vi "HapticSTM-Demod.vi"() -> ()   [LabVIEW 2019]
uses:
  Program Files/National Instruments/LabVIEW 2019/user.lib/HapticSTM/HapticSTM.lvlib
panel:
  out "Numeric":i32
  in  "Signal":u16(ring) items=["Z Val", "Demod", "AFM"]
  in  "Save":bool
  out "Origin Y":dbl
  out "Origin X":dbl
  out "Arm output":dbl
  in  "Rough adjust":dbl
  out "ZVAL":dbl
  out "Y Out":dbl
  out "X Out":dbl
  out "Max speed":dbl
  out "Width":dbl
  out "VY":dbl
  out "VZ":dbl
  out "VX":dbl
  in  "Drag":dbl=1.0
  in  "STOP":bool
  in  "START":bool
  out "Fy":dbl
  out "Fz":dbl
  out "phi":dbl
  out "psi":dbl
  out "Fx":dbl
  out "theta":dbl
  out "x":dbl
  out "y":dbl
  out "z":dbl
  in  "Fine adjust":dbl=3.5
  out "Clicks":dbl
  out "Height":dbl
  # "Sample Window"
  # "Position"
  # "Sensitivity"
  # "Force"
  # "STM I/O"
  # "Angles"
  # "Velocity"
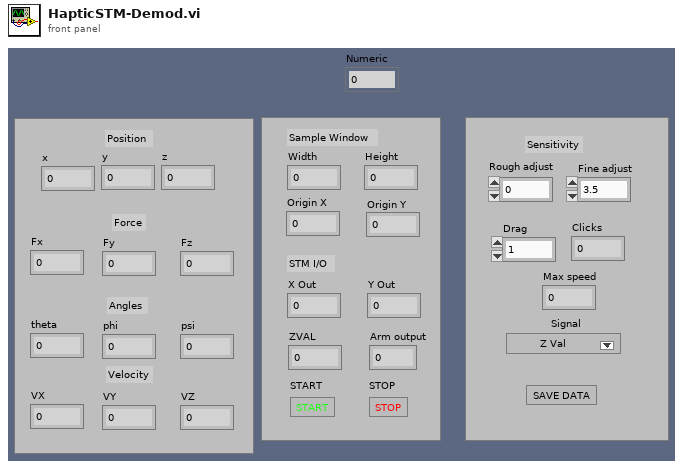
[diagram p1: front panel]
types:
  T1 = cluster{"Signal value":sgl, dbl, dbl, dbl, "Signal value":sgl}
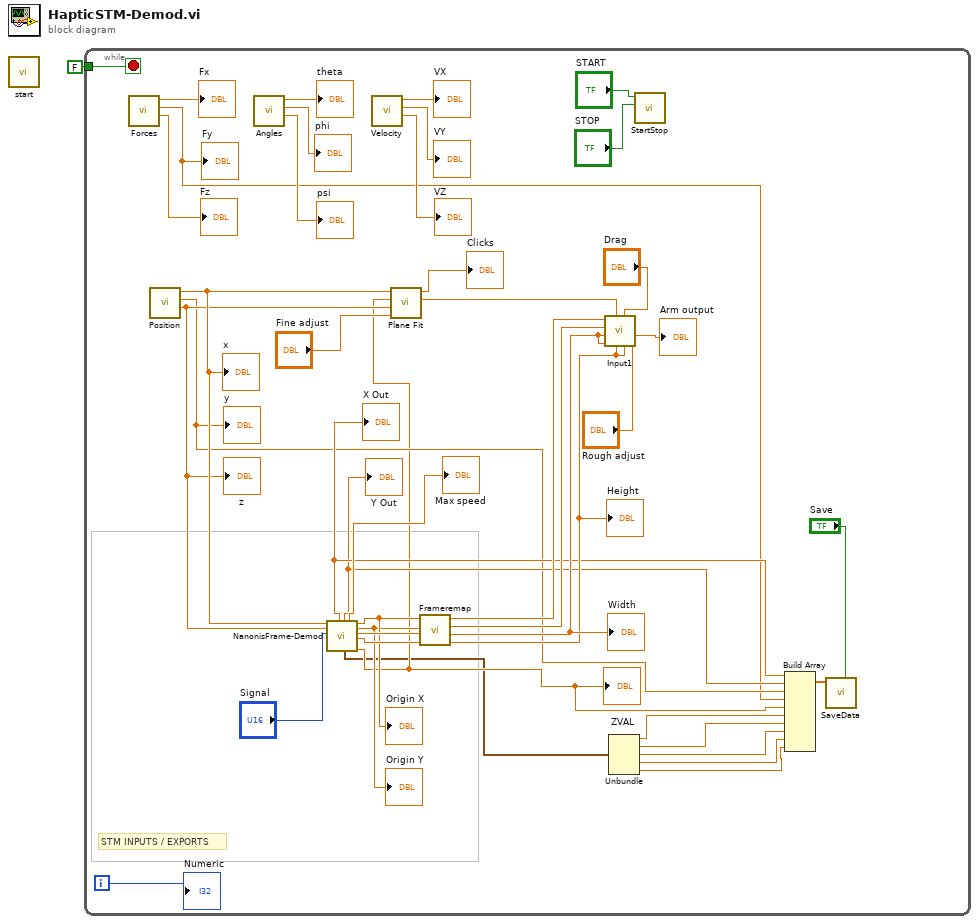
[diagram p0: block diagram]
diagram:
  n1 = call "start.vi"() -> ()  [unwired: 11 in, 1 out]
  n2 = while {
    tunnel: FALSE -> [w34]
    i -> [w3]
    stop <- w34 stop-if-true
    # "STM INPUTS / EXPORTS"
    n3 = call "Forces.vi"() -> ("Fz"=→"Fz":dbl, "Fy"=w13:dbl, "Fx"=→"Fx":dbl)  [unwired: 9 in]
    "Fy" <- w13
    n4 = call "Position.vi"() -> ("Z"=w24:dbl, "Y"=w14:dbl, "X"=w25:dbl)  [unwired: 9 in]
    "x" <- w25
    "y" <- w14
    "z" <- w24
    n5 = call "Angles.vi"() -> ("psi"=→"psi":dbl, "phi"=→"phi":dbl, "theta"=→"theta":dbl)  [unwired: 9 in]
    n6 = call "NanonisFrame-Demod.vi"("x"=w25, "z"=w24, "Signal"="Signal") -> ("X Out"=w16:dbl, "Z Out"=w15:dbl, "output cluster"=w8:T1, "Speed"=→"Max speed":dbl, "FO X"=w18:dbl, "FO Z"=w17:dbl, "FW"=w22:dbl, "FH"=w21:dbl, "CVAL (nA)"=w12:dbl)  [unwired: 8 in]
    "Y Out" <- w15
    "X Out" <- w16
    "ZVAL" <- w12
    "Origin X" <- w18
    "Origin Y" <- w17
    n7 = call "Velocity.vi"() -> ("VZ"=→"VZ":dbl, "VY"=→"VY":dbl, "VX"=→"VX":dbl)  [unwired: 9 in]
    n8 = call "Plane Fit.vi"("Sensitivity"="Fine adjust", "Z"=w24, "Nano Z"=w12, "X"=w25) -> ("Output"=w37:dbl, "Clicks"=→"Clicks":dbl)  [unwired: 6 in]
    n9 = call "Frameremap.vi"("FH"=w21, "FW"=w22, "FO Z"=w17, "FO X"=w18) -> ("FH"=w26:dbl, "FW"=w27:dbl, "Z Origin"=w35:dbl, "X Origin"=w36:dbl)  [unwired: 4 in]
    "Height" <- w26
    "Width" <- w27
    n10 = call "Input1.vi"("Current * 10^input"="Rough adjust", "Scopez"=w26, "Drag"="Drag", "FH"=w26, "Signal in"=w37, "FW"=w27, "Scopex"=w27, "Z origin"=w35, "X origin"=w36) -> ("Scaled Current"=→"Arm output":dbl)  [unwired: 2 in]
    n11 = Unbundle(w8) -> ("Signal value"=w7:sgl, w6:dbl, w5:dbl, w4:dbl, "Signal value"=w2:sgl)
    n12 = call "StartStop.vi"("STOP"="STOP", "START"="START") -> ()  [unwired: 10 in]
    n13 = Build Array(w16, w15, w14, w13, w12, w7, w6, w5, w4, w2) -> (w11:dbl[])
    n14 = call "SaveData.vi"("Save"="Save", "Data"=w11) -> ()  [unwired: 10 in]
    "Numeric" <- w3
  }
